vi "Set Data.vi"(0 "2D String Logging Data in":refnum<class "2D String Logging Data.lvclass">, 5 "Group Name":string, 7 "Channel Names":string[](array[string]), 9 "Data":string[][](array[string]), 11 "error in (no error)":errorcluster) -> (4 "2D String Logging Data out":refnum<class "2D String Logging Data.lvclass">, 15 "error out":errorcluster)   [LabVIEW 2024, in "Logging Data.lvlib" / "2D String Logging Data.lvclass"]
uses:
  2D String Logging Data.lvclass
  2D String Logging Data.lvclass/2D String Logging Data.ctl
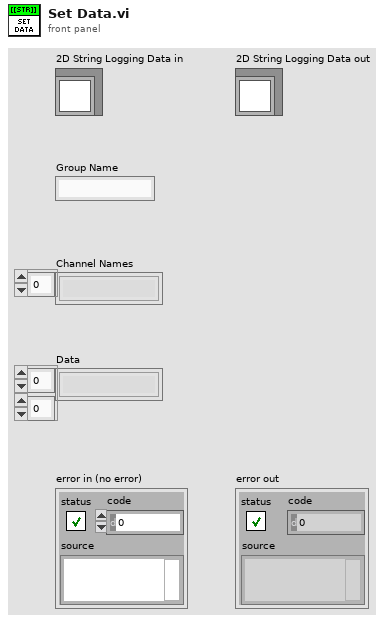
[diagram p1: front panel]
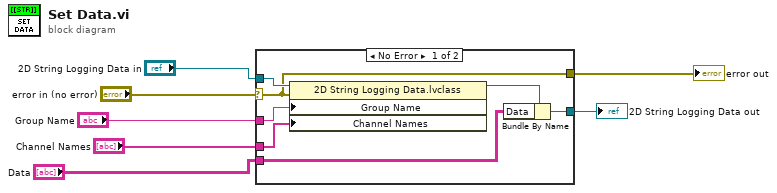
[diagram p0: block diagram]
diagram:
  n1 = case shown="No Error" "error in (no error)" {
    selector: "error in (no error)" -> [w13 w16]
    tunnel: [w13 w16] -> w6
    tunnel: [w11 w15] -> w4
    tunnel: "2D String Logging Data in" -> [w14 w15]
    tunnel: "Group Name" -> [w9 _]
    tunnel: "Channel Names" -> [w8 _]
    tunnel: "Data" -> [w10 _]
    frame No Error {
      n2 = property class="2D String Logging Data.lvclass"(reference=w14, error in=w13, "Group Name"=w9, "Channel Names"=w8) -> (reference out=w12:refnum<class "2D String Logging Data.lvclass">)  [unwired: 1 out]
      n3 = Bundle By Name(cluster=w12, "Data"=w10) -> (w11:refnum<class "2D String Logging Data.lvclass">)
    }
    frame Error {
    }
  }
  "error out" <- w6
  "2D String Logging Data out" <- w4
